vi "Read Attributes.vi"(11 "Set DER SetPointPF Msg":refnum<class "Set DER SetPointPF Msg.lvclass">) -> (2 "Payload":cluster{"DER_SetPointPF":T1})   [LabVIEW 2018, in "Device Communication and Control Abstract Actor.lvlib" / "Set DER SetPointPF Msg.lvclass"]
uses:
  Set DER SetPointPF Msg.lvclass
  <vilib>/ORNL/CSEISMIC DDS/CSEISMIC DDS Base/Data Types/DER_SetPointPF.ctl
  <vilib>/ORNL/CSEISMIC DDS/CSEISMIC DDS Base/Data Types/Controls/DeviceID.ctl
  Set DER SetPointPF Msg.lvclass/Set DER SetPointPF Msg.ctl
  <vilib>/ORNL/CSEISMIC DDS/CSEISMIC DDS Base/CSEISMIC DDS.lvclass
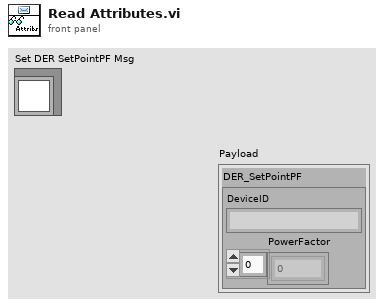
[diagram p1: front panel]
types:
  T1 = typedef "CSEISMIC DDS.lvlib/CSEISMIC DDS.lvclass/DER_SetPointPF.ctl" = cluster{"DeviceID":T2, "PowerFactor":dbl[]}
  T2 = typedef "CSEISMIC DDS.lvlib/CSEISMIC DDS.lvclass/DeviceID.ctl" = string
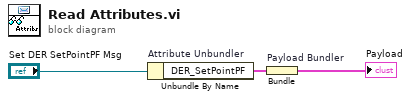
[diagram p0: block diagram]
diagram:
  n1 = Unbundle By Name "Attribute Unbundler"("Set DER SetPointPF Msg") -> ("DER_SetPointPF"=w1:T1)
  n2 = Bundle "Payload Bundler"("DER_SetPointPF"=w1) -> (→"Payload":cluster{"DER_SetPointPF":T1})  [unwired: 1 in]
